vi "get c8 peak sub.vi"(10 "laser task in":refnum<k21>, 11 "germanium task in":refnum<k21>) -> (0 "lower limit":dbl, 1 "upper limit":dbl, 2 "laser task out":refnum<k21>, 3 "germanium task out":refnum<k21>)   [LabVIEW 2018]
uses:
  <vilib>/DAQmx/write.llb/DAQmx Write (Analog DBL 1Chan 1Samp).vi
  b68e9a59-4eba-4379-9156-84f4316a9dab.vi
  <vilib>/DAQmx/read.llb/DAQmx Read (Analog DBL 1Chan 1Samp).vi
  <vilib>/Analysis/baseanly.llb/Mean (DBL).vi
  <vilib>/DAQmx/miscellaneous.llb/DAQmx Fill In Error Info.vi
  <vilib>/ptbypt/NI_PtbyPt.lvlib
  <vilib>/Analysis/NI_AALBase.lvlib
  <vilib>/Analysis/NI_AAL_SigProc.lvlib
panel:
  out "c8 peak (V)":dbl
  in  "sample length":i32=100
  in  "step length (seconds)":dbl=1.0
  out "laser voltage":dbl
  out "diode voltage":dbl
  out "Waveform Chart":cluster{"mean":dbl, "start voltage":dbl}(graph)
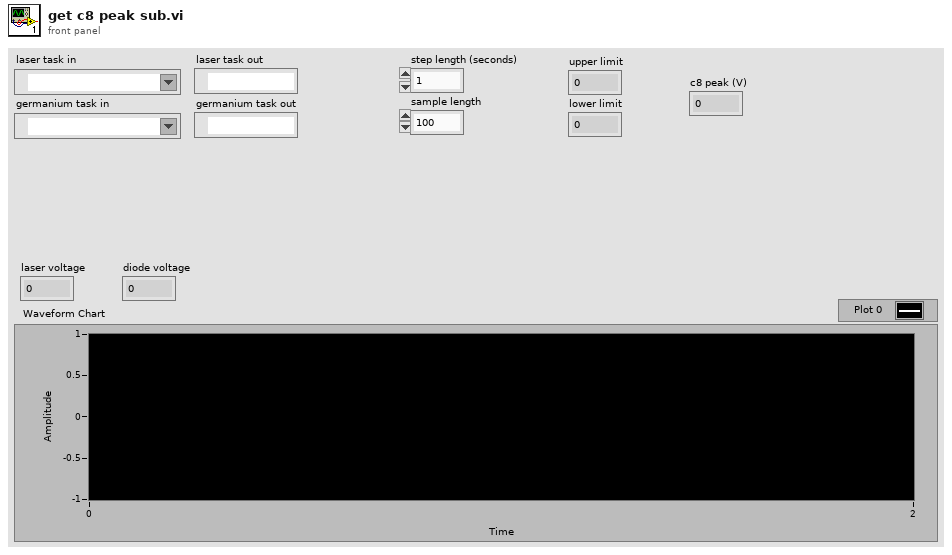
[diagram p1: front panel]
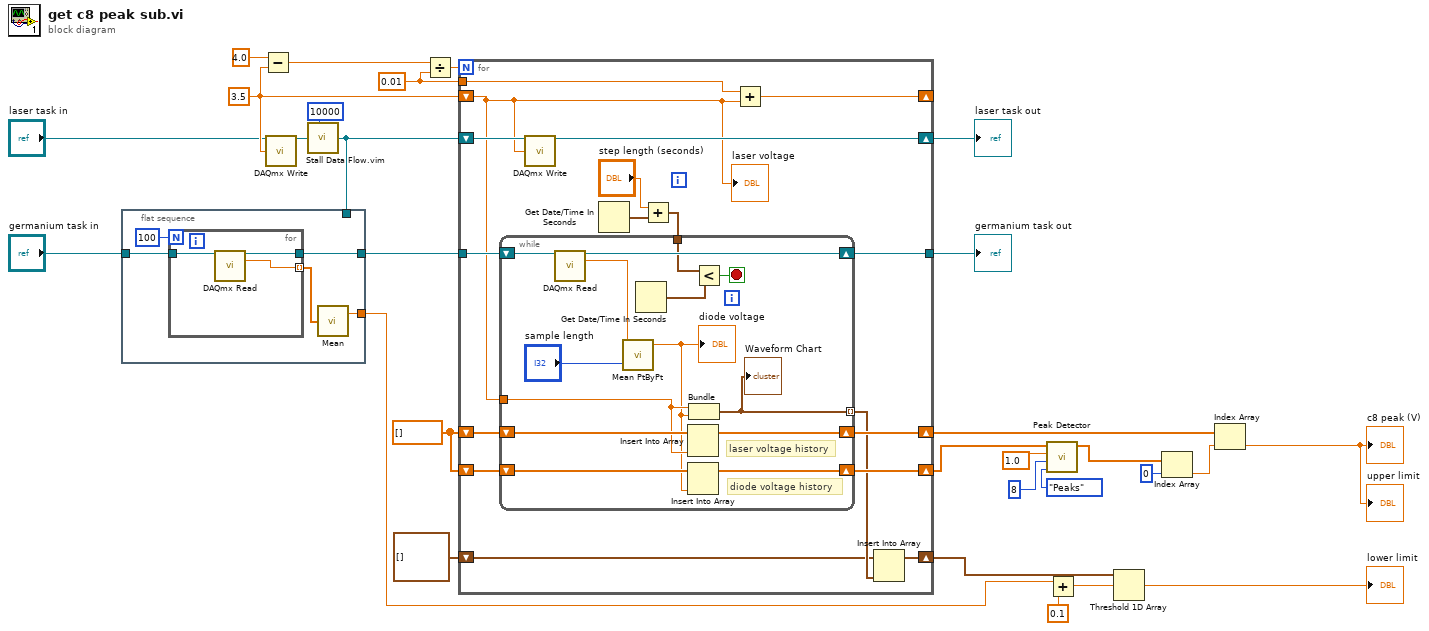
[diagram p0: block diagram]
diagram:
  w23 = 0.01 ("step size")
  w26 = 3.5 ("start voltage")
  w16 = dbl[] []
  n1 = flat-sequence {
    tunnel: "germanium task in" -> [w34]
    tunnel: [w33] -> w18
    tunnel: w17 -> [_]
    tunnel: [w30] -> w3
    frame #0 {
      n2 = for {
        N: 100 -> [_]
        tunnel: [w35] -> w31 mode=indexing
        tunnel: w34 -> [w37]
        tunnel: [w36] -> w33
        n3 = call-poly <vilib>:"DAQmx Read.vi"("task/channels in"=w37) -> ("task out"=w36:refnum<k21>, "data"=w35:dbl)  [unwired: 12 in, 1 out]
      }
      n4 = call-poly <vilib>:"Mean.vi"("X"=w31) -> ("mean"=w30:dbl)  [unwired: 1 out]
    }
  }
  n5 = Subtract(x=4.0 ("end voltage"), y=w26) -> (x-y=w25:dbl)
  n6 = call-poly <vilib>:"DAQmx Write.vi"("task/channels in"="laser task in", "data"=w26) -> ("task out"=w29:refnum<k21>)  [unwired: 11 in, 2 out]
  n7 = call "Stall Data Flow.vim"("value in"=w29, "milliseconds to wait"=u32 10000) -> ("value out"=w17:refnum<k21>)  [unwired: 1 out]
  n8 = Divide(x=w25, y=w23) -> (x/y=w24:dbl)
  n9 = for {
    N: w24 -> [_]
    shift-right: [w51] -> w21
    shift-left: w17 -> [w54]
    shift-right: [w53] -> _
    shift-left: w26 -> [w48]
    tunnel: w23 -> [w52]
    tunnel: w18 -> [w50]
    tunnel: [w49] -> w20
    shift-right: [w46] -> w6
    shift-left: w16 -> [w47]
    shift-right: [w44] -> w5
    shift-left: w16 -> [w45]
    shift-right: [w42] -> w4
    shift-left: cluster{"start voltage":dbl, "mean":dbl}[] [] -> [w41]
    n10 = call-poly <vilib>:"DAQmx Write.vi"("task/channels in"=w54, "data"=w48) -> ("task out"=w51:refnum<k21>)  [unwired: 11 in, 2 out]
    n11 = Get Date/Time In Seconds() -> (seconds since 1Jan1904=w39:timestamp)
    n12 = Add(x="step length (seconds)", y=w39) -> (x+y=w38:timestamp)
    n13 = while {
      shift-right: [w67] -> w49
      shift-left: w50 -> [w68]
      tunnel: w48 -> [w58]
      shift-right: [w61] -> w46
      shift-left: w47 -> [w62]
      shift-right: [w59] -> w44
      shift-left: w45 -> [w60]
      tunnel: [w56] -> w43 mode=indexing
      tunnel: w38 -> [w55]
      stop <- w64 stop-if-true
      # "laser voltage history"
      # "diode voltage history"
      n14 = call-poly <vilib>:"DAQmx Read.vi"("task/channels in"=w68) -> ("task out"=w67:refnum<k21>, "data"=w65:dbl)  [unwired: 12 in, 1 out]
      n15 = call <vilib>:"Mean PtByPt.vi"("x"=w65, "sample length"="sample length") -> ("mean"=w57:dbl)  [unwired: 2 in, 1 out]
      "diode voltage" <- w57
      n16 = Get Date/Time In Seconds() -> (seconds since 1Jan1904=w63:timestamp)
      n17 = Insert Into Array(array=w62, new element=w58) -> (w61:dbl[])  [unwired: 1 in]
      n18 = Insert Into Array(array=w60, new element=w57) -> (w59:dbl[])  [unwired: 1 in]
      n19 = Bundle("start voltage"=w58, "mean"=w57) -> (w56:cluster{"start voltage":dbl, "mean":dbl})  [unwired: 1 in]
      "Waveform Chart" <- w56
      n20 = Less?(x=w55, y=w63) -> (x < y?=w64:bool)
    }
    n21 = Add(x=w52, y=w48) -> (x+y=w53:dbl)
    n22 = Insert Into Array(array=w41, new element=w43) -> (w42:cluster{"start voltage":dbl, "mean":dbl}[])  [unwired: 1 in]
    "laser voltage" <- w48
  }
  "laser task out" <- w21
  "germanium task out" <- w20
  n23 = call <vilib>:"Peak Detector.vi"("peaks/valleys"=enum32{"Peaks", "Valleys"}."Peaks", "width"=8, "threshold"=1.0, "X"=w5) -> ("Locations"=w12:dbl[])  [unwired: 3 in, 4 out]
  n24 = Add(x=w3, y=0.1) -> (x+y=w8:dbl)
  n25 = Threshold 1D Array(2:w8, 3:w4) -> (0:→"lower limit":dbl)  [unwired: 1 in]
  n26 = Index Array(array=w12, index=0) -> (element=w10:dbl)
  n27 = Index Array(array=w6, index=w10) -> (element=→"c8 peak (V)" →"upper limit":dbl)
